vi "TestUplink Addon.vi"(0 "RFSA Handle In":refnum<k15>, 1 "SMU Handle In":refnum<k15>, 2 "FPGA VI Reference In":refnum<k20>, 3 "UL Rx Timeout":i64, 5 "Enum":T1, 6 "Resp Timeout (ms)":i32, 7 "error in (no error)":errorcluster, 8 "UL Rx Central Freq":i64, 9 "DxSupply":string="2", 10 "UL Data Rate":i64, 11 "Pwr Reduction (dB/2)":i8=1, 12 "UL Rx Span":i64, 14 "Test Mode":i8=1) -> (13 "Timeout Flag":bool=TRUE, 15 "Set Freq Offset OK":bool, 19 "String":string, 22 "UL Rx Payload":string, 23 "Meas UL Rx Freq":i64, 24 "Meas UL Idd":dbl, 27 "error out":errorcluster)   [LabVIEW 2018]
uses:
  Resources_Test/UART/ControlTestSlot.ctl
  <vilib>/Analysis/4window.llb/windowTd.ctl
  <vilib>/measure/maspectr.llb/FFT Power Spectrum and PSD for 1 Chan (CDB).vi
  <vilib>/Analysis/NI_AALPro.lvlib
  SigFox 2015 - Monarch/RFSA e RFGA/SigFox Test.lvlib
  <vilib>/measure/NI_MAPro.lvlib
panel:
  out "Length Indicator (Binary)":string
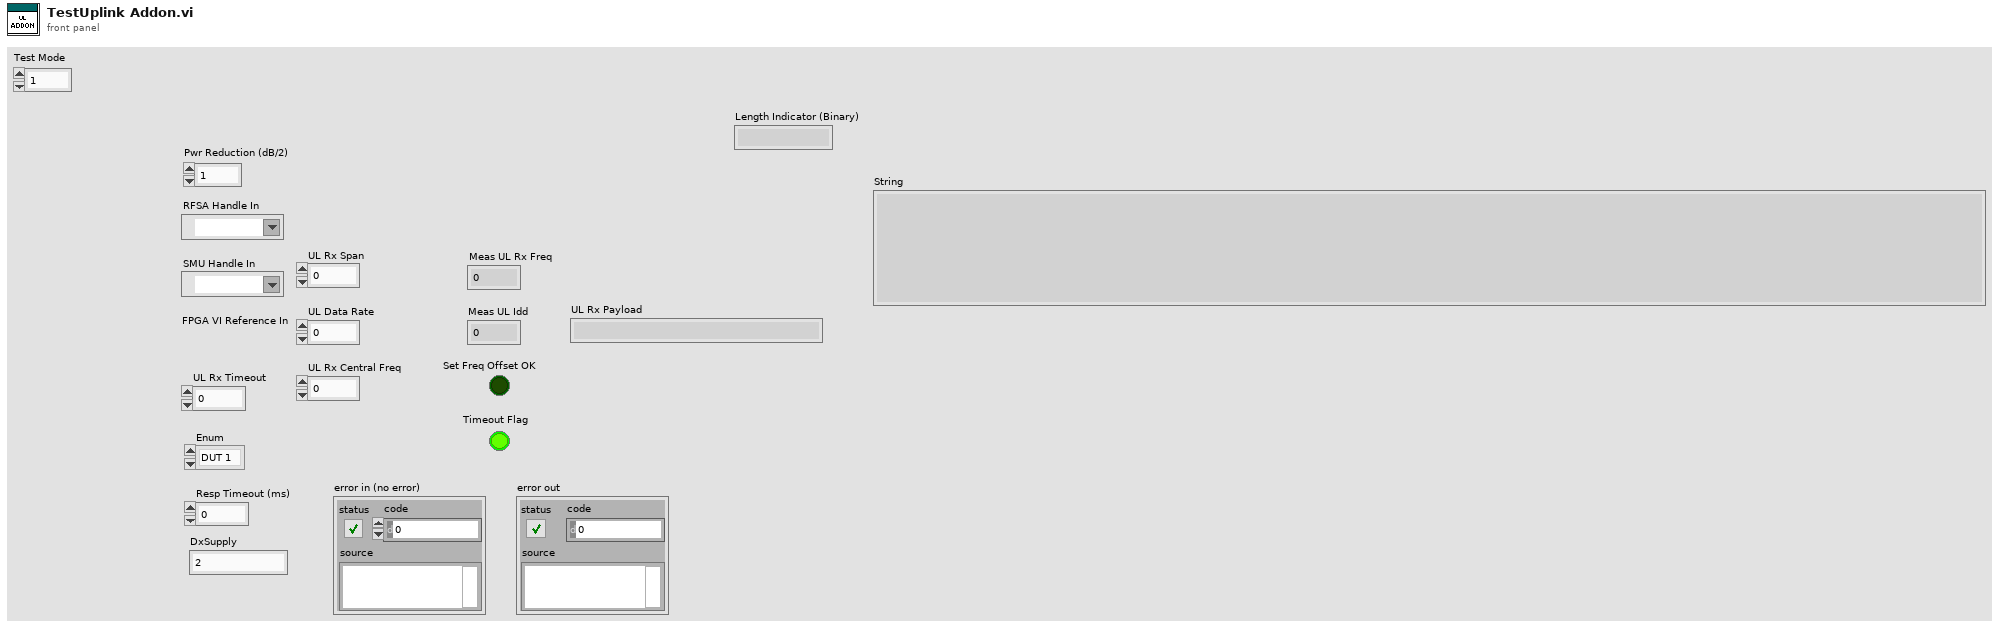
[diagram p1: front panel]
types:
  T1 = typedef "ControlTestSlot.ctl" = enum16{"DUT 1", "DUT 2"}
  T2 = cluster{"averaging mode":enum16{"No averaging", "Vector averaging", "RMS averaging", "Peak hold"}, "weighting mode":enum16{"Linear", "Exponential"}, "number of averages":u32}
  T3 = enum16{"0", "1", "2", "3", "4", "5", "6", "7", "8", "9", "10", "11", "12"}
  T4 = typedef "NI_AALPro.lvlib/windowTd.ctl" = u32
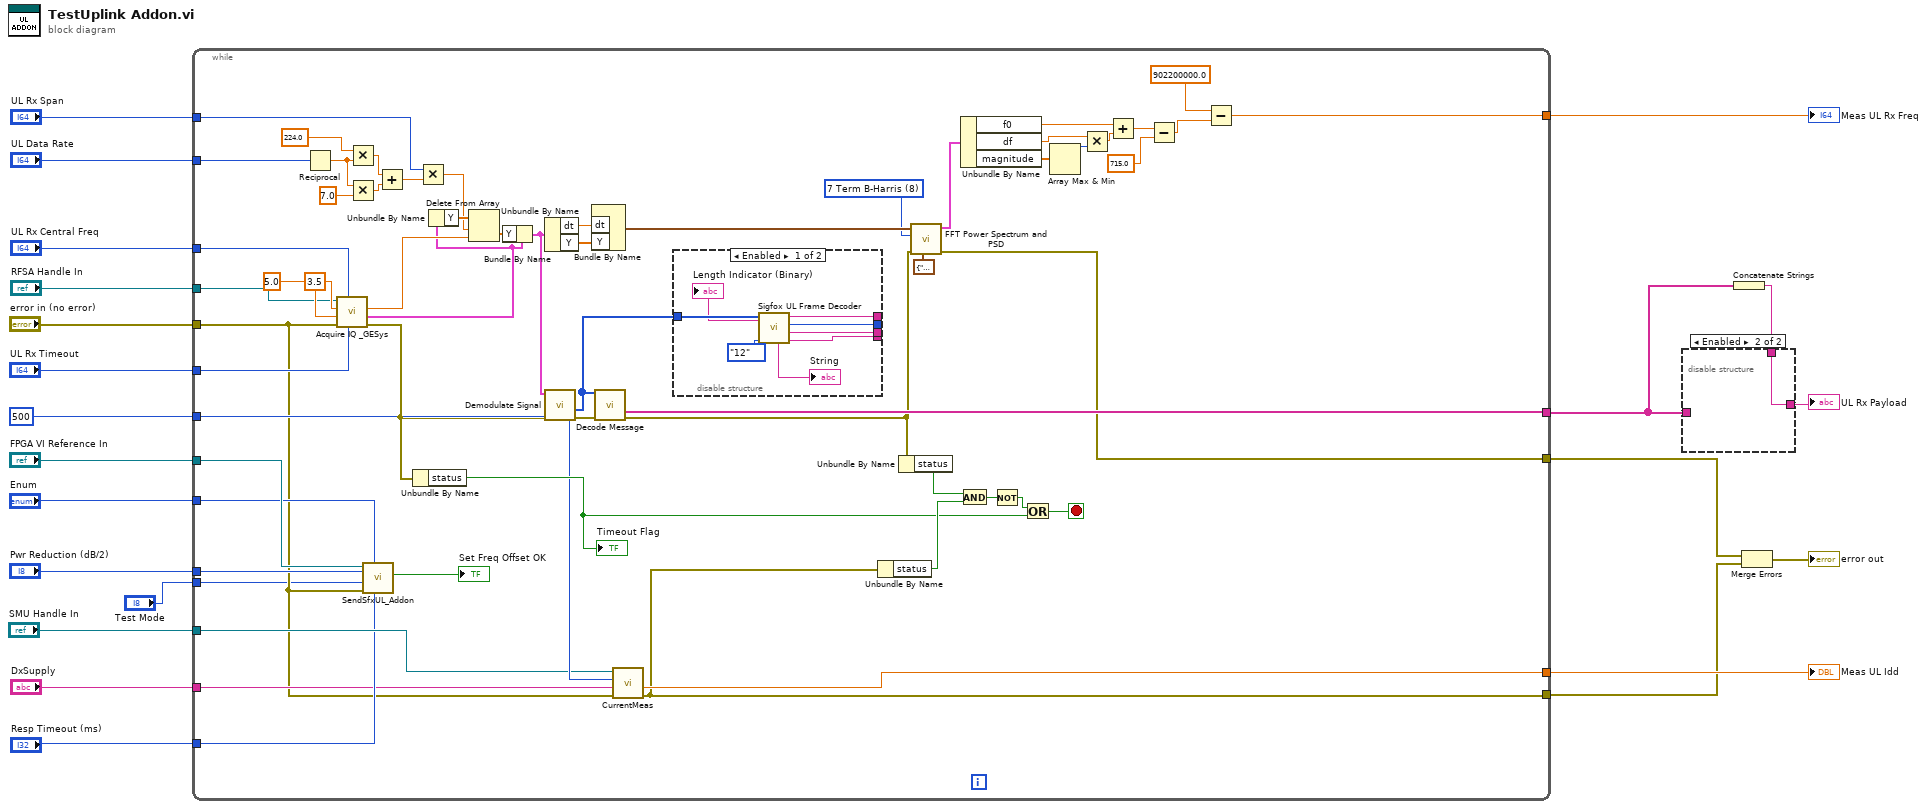
[diagram p0: block diagram]
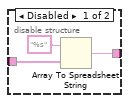
[diagram p2: hidden frame]
diagram:
  n1 = while {
    tunnel: [w80] -> w3
    tunnel: [w67] -> w8
    tunnel: 500 ("Measure Record Length") -> [w69]
    tunnel: [w77] -> w10
    tunnel: "UL Rx Timeout" -> [w70]
    tunnel: "Resp Timeout (ms)" -> [w33]
    tunnel: "Enum" -> [w31]
    tunnel: "UL Rx Central Freq" -> [w65]
    tunnel: "UL Rx Span" -> [w34]
    tunnel: "SMU Handle In" -> [w68]
    tunnel: "RFSA Handle In" -> [w66]
    tunnel: "UL Data Rate" -> [w55]
    tunnel: [w38] -> w5
    tunnel: "FPGA VI Reference In" -> [w32]
    tunnel: "DxSupply" -> [w29]
    tunnel: "error in (no error)" -> [w26]
    tunnel: [w40] -> w12
    tunnel: "Pwr Reduction (dB/2)" -> [w27]
    tunnel: "Test Mode" -> [w23]
    stop <- w73 stop-if-true
    w42 = T4 8 items=["Rectangle"=0, "Hanning"=1, "Hamming"=2, "Blackman-Harris"=3, "Exact Blackman"=4, "Blackman"=5, "Flat Top"=6, "4 Term B-Harris "=7, "7 Term B-Harris"=8, "Low Sidelobe"=9, "Blackman Nuttall"=11, "Triangle"=30, "Bartlett-Hanning"=31, "Bohman"=32, "Parzen"=33, "Welch"=34, "Kaiser"=60, "Dolph-Chebyshev"=61, "Gaussian"=62] ("window")
    n2 = Reciprocal(x=w55) -> (1/x=w61:dbl)
    n3 = call "Acquire IQ _GESys.vi"("timeout (10 sec)"=w70, "Carrier Frequency (Hz)"=w65, "error in (no error)"=w26, "Reference Position (%)"=5.0, "Burst Length (sec)"=3.5, "instrument handle"=w66) -> ("error out"=w64:errorcluster, "IQ"=w28:cluster{"t0":dbl, "dt":dbl, "Y":cdb[]}, "Pre-Trigger"=w54:dbl)  [unwired: 2 in, 1 out]
    n4 = Multiply(x=224.0, y=w61) -> (x*y=w58:dbl)
    n5 = Multiply(x=w61, y=7.0) -> (x*y=w57:dbl)
    n6 = call "SendSfxUL_Addon.vi"("Resp Timeout (ms)"=w33, "Active Dut"=w31, "Error In"=w26, "Test Mode"=w23, "Pwr Reduction (dB/2)"=w27, "FPGA Reference"=w32) -> ("Tx Testmode OK"=→"Set Freq Offset OK":bool)  [unwired: 1 in, 4 out]
    n7 = Add(x=w58, y=w57) -> (x+y=w59:dbl)
    n8 = Unbundle By Name(w64) -> ("status"=w71:bool)
    "Timeout Flag" <- w71
    n9 = Multiply(x=w34, y=w59) -> (x*y=w56:dbl)
    n10 = Unbundle By Name(w28) -> ("Y"=w63:cdb[])
    n11 = Delete From Array(array=w63, length=w56, index=w54) -> (deleted portion=w53:cdb[])  [unwired: 1 out]
    n12 = Bundle By Name(cluster=w28, "Y"=w53) -> (w24:cluster{"t0":dbl, "dt":dbl, "Y":cdb[]})
    n13 = Unbundle By Name(w24) -> ("dt"=w52:dbl, "Y"=w51:cdb[])
    n14 = call "Demodulate Signal.vi"("error in (no error)"=w64, "Complex Waveform"=w24) -> ("error out"=w81:errorcluster, "Output bit stream"=w25:i8[])  [unwired: 6 in, 2 out]
    n15 = Bundle By Name("dt"=w52, "Y"=w51) -> (w50:waveform(cdb))  [unwired: 1 in]
    n16 = call "Decode Message.vi"("Bit Stream"=w25, "error in"=w81) -> ("Payload"=w80:string[], "error out"=w41:errorcluster)  [unwired: 8 in, 4 out]
    n17 = call "CurrentMeas.vi"("error in (no error)"=w26, "DxSupply"=w29, "Measure Record Length"=w69, "instrument handle"=w68) -> ("error out"=w67:errorcluster, "Idd Peak"=w77:dbl)  [unwired: 4 in, 2 out]
    n18 = disable-structure shown="Enabled" {
      disable-tunnel: w25 -> [w89 _]
      disable-tunnel: [w87 _] -> _
      disable-tunnel: [w86 _] -> _
      disable-tunnel: [w85 _] -> _
      disable-tunnel: [w84 _] -> _
      frame Enabled {
        n19 = call "Sigfox UL Frame Decoder.vi"("Payload Size (Bytes)"=T3."12", "UL Frame"=w89) -> ("Payload (Hex)"=w87:string, "ID (Hex)"=w86:string, "Message Counter"=w85:u16, "BF + REP (Binary)"=w84:string, "String"=→"String":string, "Length Indicator (Binary)"=→"Length Indicator (Binary)":string)  [unwired: 4 in]
      }
      frame Disabled {
      }
    }
    n20 = Unbundle By Name(w67) -> ("status"=w75:bool)
    n21 = Unbundle By Name(w41) -> ("status"=w76:bool)
    n22 = call-poly <vilib>:"FFT Power Spectrum and PSD.vi"("averaging parameters"=T2 {"averaging mode"=enum."Peak hold", "weighting mode"=enum."Exponential", "number of averages"=8}, "error in (no error)"=w41, "window"=w42, "time signal"=w50) -> ("error out"=w40:errorcluster, "Power Spectrum / PSD"=w49:cluster{"f0":dbl, "df":dbl, "magnitude":dbl[]})  [unwired: 4 in, 2 out]
    n23 = And(x=w76, y=w75) -> (x .and. y?=w74:bool)
    n24 = Unbundle By Name(w49) -> ("f0"=w47:dbl, "df"=w45:dbl, "magnitude"=w48:dbl[])
    n25 = Not(x=w74) -> (.not. x?=w72:bool)
    n26 = Or(x=w72, y=w71) -> (x .or. y?=w73:bool)
    n27 = Array Max & Min(array=w48) -> (max index (indices)=w44:i32)  [unwired: 3 out]
    n28 = Multiply(x=w45, y=w44) -> (x*y=w46:dbl)
    n29 = Add(x=w47, y=w46) -> (x+y=w37:dbl)
    n30 = Subtract(x=w37, y=715.0) -> (x-y=w36:dbl)
    n31 = Subtract(x=902200000.0, y=w36) -> (x-y=w38:dbl)
  }
  "Meas UL Idd" <- w10
  "Meas UL Rx Freq" <- w5
  n32 = Concatenate Strings(w3) -> (w2:string)
  n33 = disable-structure shown="Enabled" {
    disable-tunnel: [w91 w93] -> w6
    disable-tunnel: w3 -> [w90 _]
    disable-tunnel: w2 -> [_ w93]
    frame Disabled {
      n34 = Array To Spreadsheet String(array=w90, 3:"%s" ("format string")) -> (spreadsheet string=w91:string)  [unwired: 1 in]
    }
    frame Enabled {
    }
  }
  "UL Rx Payload" <- w6
  n35 = Merge Errors(w12, w8) -> (→"error out":errorcluster)
